vi "Build Messgenger.vi"(4 "Paras In 2":variant, 6 "Paras In":variant, 7 "SMGQ Messenger Factory in":refnum<class "Simple Map Group Queue Messenger Factory.lvclass">, 8 "error in (no error)":errorcluster, 10 "Root Actor In":refnum<class "Root Actor.lvclass">, 11 "System Modules Factory In":refnum<class "System Modules Factory.lvclass">) -> (0 "error out":errorcluster, 2 "Root Actor Out":refnum<class "Root Actor.lvclass">, 3 "System Modules Factory Out":refnum<class "System Modules Factory.lvclass">, 5 "SMGQ Messenger Factory out":refnum<class "Simple Map Group Queue Messenger Factory.lvclass">)   [LabVIEW 2024, in "Simple Map Group Queue Messenger Factory.lvclass"]
uses:
  Simple Map Group Queue Messenger Factory.lvclass
  Ancestor Class/Actor/Root Actor/Root Actor.lvclass
  Ancestor Class/Factory/System Modules Factory/System Modules Factory.lvclass
  Ancestor Class/Message/Message.lvclass
  Messenger/Simple Map Queue Group Messenger/Simple Map Queue Group Messenger.lvclass
  Ancestor Class/Actor/System Actor/System Actor.lvclass/System Actor.ctl
  Ancestor Class/Factory/System Modules Factory/System Modules Factory.lvclass/System Modules Factory.ctl
  Ancestor Class/Factory/System Modules Factory/Public Data/Read System Module ID.vi
  Ancestor Class/Actor/System Actor/Public Data/Read ID.vi
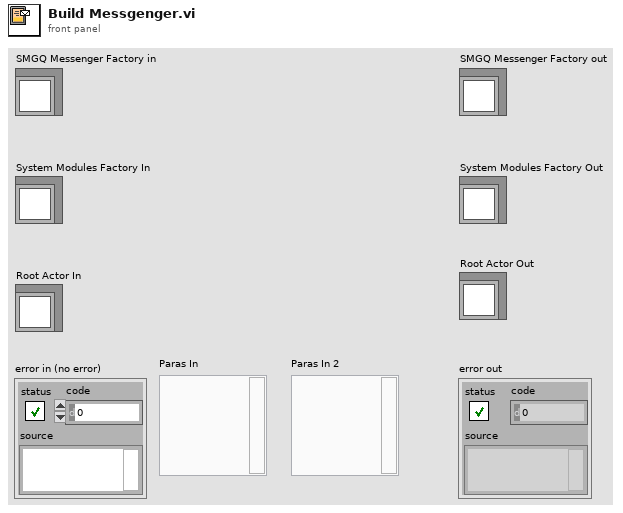
[diagram p1: front panel]
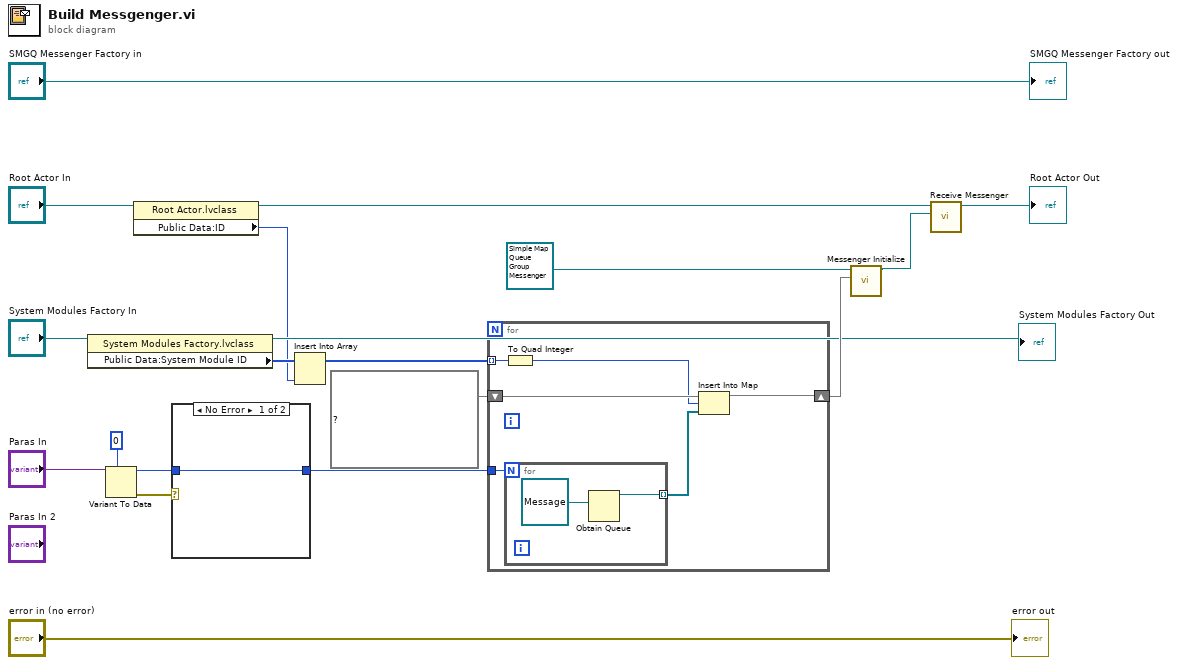
[diagram p0: block diagram]
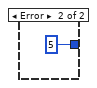
[diagram p2: hidden frame]
diagram:
  n1 = property class="System Modules Factory.lvclass"(reference="System Modules Factory In") -> (reference out=→"System Modules Factory Out":refnum<class "System Modules Factory.lvclass">, "Public Data:System Module ID"=w3:i64[])  [unwired: 1 in, 1 out]
  n2 = Variant To Data(type=0, Variant="Paras In") -> (data=w8:i32, error out=w9:errorcluster)  [unwired: 1 in]
  n3 = property class="Root Actor.lvclass"(reference="Root Actor In") -> (reference out=w4:refnum<class "Root Actor.lvclass">, "Public Data:ID"=w1:i64)  [unwired: 1 in, 1 out]
  n4 = case shown="No Error" w9 {
    tunnel: w8 -> [w20 _]
    tunnel: [w20 5] -> w7
    frame No Error {
    }
    frame Error {
    }
  }
  n5 = Insert Into Array(array=w3, new element=w1) -> (w2:i64[])  [unwired: 1 in]
  n6 = for {
    tunnel: w2 -> [w25] mode=indexing
    shift-right: [w26] -> w13
    shift-left: map{i64, refnum<queue>[]} {} ("Child Nodes") -> [w27]
    tunnel: w7 -> [w23]
    n7 = To Quad Integer(1:w25) -> (0:w24:i64)
    n8 = for {
      N: w23 -> [_]
      tunnel: [w28] -> w22 mode=indexing
      n9 = Obtain Queue(element data type=refnum<class "Message.lvclass"> refnum ("Message.lvclass")) -> (queue out=w28:refnum<queue>)  [unwired: 4 in, 2 out]
    }
    n10 = Insert Into Map(map in=w27, key=w24, value=w22) -> (map out=w26:map{i64, refnum<queue>[]})  [unwired: 2 out]
  }
  n11 = call-dynamic "Messenger Initialize.vi"("Paras In"=w13, "Simple Map Queue Group Messenger in"=refnum<class "Simple Map Queue Group Messenger.lvclass"> refnum ("Simple Map Queue Group Messenger.lvclass")) -> ("Simple Map Queue Group Messenger out"=w12:refnum<class "Simple Map Queue Group Messenger.lvclass">)  [unwired: 8 in, 1 out]
  n12 = call-dynamic "Receive Messenger.vi"("Messenger In"=w12, "Root Actor in"=w4) -> ("Root Actor out"=→"Root Actor Out":refnum<class "Root Actor.lvclass">)  [unwired: 8 in, 1 out]
  "error out" <- "error in (no error)"
  "SMGQ Messenger Factory out" <- "SMGQ Messenger Factory in"
